vi "HaloDrive.vi"(0 "RobotDriveDevRef 2":T1={"DevStatus"={"status"=FALSE, "code"=0, "source"=""}, "Motors[]"=[], "Square Inputs"=FALSE, "Max Output"=1.0}, 1 "QwikTurnButton":bool, 5 "Left axis value":dbl, 9 "Right axis value":dbl, 11 "error in (no error)":errorcluster, 12 "Sensitivity":dbl) -> (4 "RobotDriveDevRef":T1={"DevStatus"={"status"=FALSE, "code"=0, "source"=""}, "Motors[]"=[], "Square Inputs"=FALSE, "Max Output"=1.0}, 6 "Motor Values":dbl[](array[numeric]), 8 "Left Output":dbl, 10 "Right Output":dbl, 15 "error out":errorcluster)   [LabVIEW 2015]
uses:
  <vilib>/Rock Robotics/WPI/RobotDrive/WPI_RobotDriveDevRef.ctl
  <vilib>/Rock Robotics/WPI/MotorControl/WPI_MotorControlDeviceRef.ctl
  <vilib>/Rock Robotics/WPI/MotorControl/WPI_MotorControlType.ctl
  <vilib>/Rock Robotics/SystemInterfaces/DIO/FPGA_DIOPWMChannel.ctl
  <vilib>/Rock Robotics/WPI/PWM/WPI_PWMDeadband.ctl
  <vilib>/Rock Robotics/WPI/CAN/Jaguar/SubVIs/WPI_CANJaguar_ControlMode.ctl
  <vilib>/Rock Robotics/WPI/CAN/TalonSRX/WPI_CANTalonSRX_APIControlMode.ctl
  <vilib>/Rock Robotics/SystemInterfaces/NetworkCommunication/NetComm_UsageReport_ResourceType.ctl
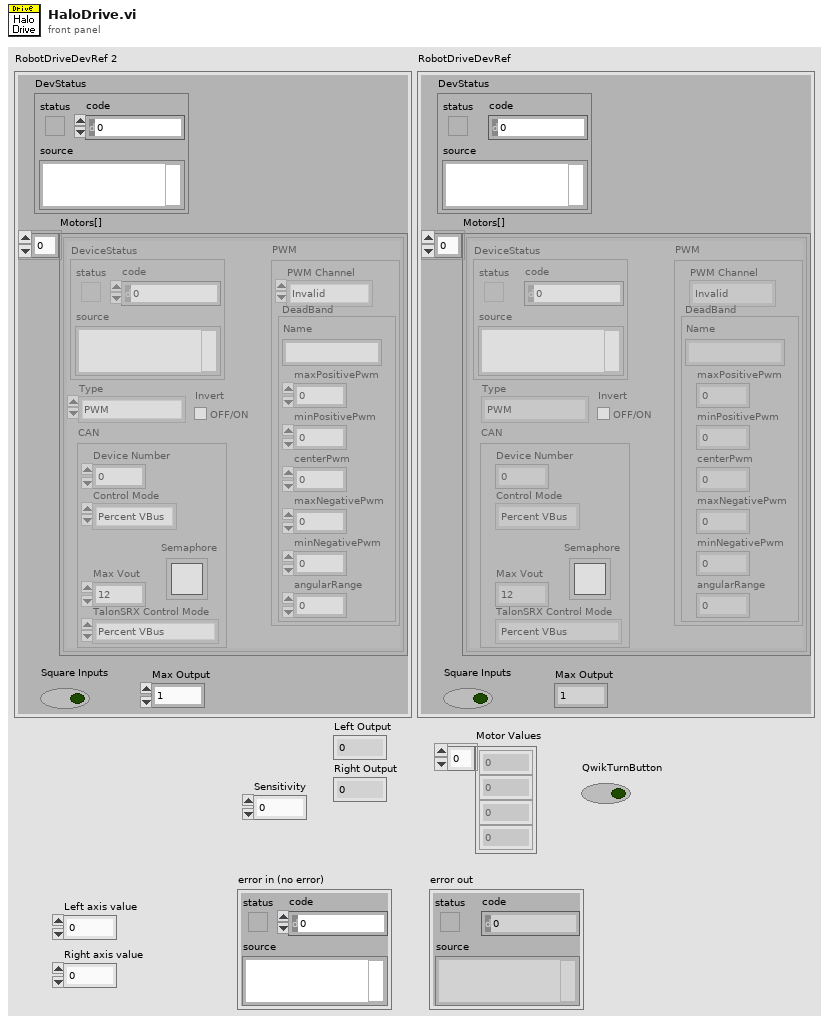
[diagram p1: front panel]
types:
  T1 = typedef "WPI_RobotDriveDevRef.ctl" = cluster{"DevStatus":errorcluster, "Motors[]":T2[], "Square Inputs":bool, "Max Output":dbl}
  T2 = typedef "WPI_MotorControlDeviceRef.ctl" = cluster{"DeviceStatus":errorcluster, "Type":T3, "PWM":cluster{"PWM Channel":T4, "DeadBand":T5}, "CAN":cluster{"Device Number":u8, "Control Mode":T6, "Semaphore":T7, "Max Vout":dbl, "TalonSRX Control Mode":T8}, "Invert":bool}
  T3 = typedef "WPI_MotorControlType.ctl" = enum16{"PWM", "CAN", "CANTalonSRX"}
  T4 = typedef "FPGA_DIOPWMChannel.ctl" = enum8{"PWM 0", "PWM 1", "PWM 2", "PWM 3", "PWM 4", "PWM 5", "PWM 6", "PWM 7", "PWM 8", "PWM 9", "PWM MXP 0", "PWM MXP 1", "PWM MXP 2", "PWM MXP 3", "PWM MXP 4", "PWM MXP 5", "PWM MXP 6", "PWM MXP 7", "PWM MXP 8", "PWM MXP 9", "Invalid"}
  T5 = typedef "WPI_PWMDeadband.ctl" = cluster{"Name":string, "maxPositivePwm":i32, "minPositivePwm":i32, "centerPwm":i32, "maxNegativePwm":i32, "minNegativePwm":i32, "angularRange":u16}
  T6 = typedef "WPI_CANJaguar_ControlMode.ctl" = enum8{"Percent VBus", "Current", "Speed", "Position", "Voltage"}
  T7 = typedef "Semaphore RefNum" = refnum<k1>
  T8 = typedef "WPI_CANTalonSRX_APIControlMode.ctl" = enum8{"Percent VBus", "Speed", "Position", "Slave", "Unchanged / Invalid", "Voltage Compensation", "Current", "Motion Profile"}
  T9 = typedef "NetComm_UsageReport_ResourceType.ctl" = enum8{"Controller", "Module", "Language", "CANPlugin", "Accelerometer", "ADXL345", "AnalogChannel", "AnalogTrigger", "AnalogTriggerOutput", "CANJaguar", "Compressor", "Counter", "Dashboard", "DigitalInput", "DigitalOutput", "DriverStationCIO", "DriverStationEIO", "DriverStationLCD", "Encoder", "GearTooth", "Gyro", "I2C", "Framework", "Jaguar", "Joystick", "Kinect", "KinectStick", "PIDController", "Preferences", "PWM", "Relay", "RobotDrive", "SerialPort", "Servo", "Solenoid", "SPI", "Task", "Ultrasonic", "Victor", "Button", "Command", "AxisCamera", "PCVideoServer", "SmartDashboard", "Talon", "HiTechnicColorSensor", "HiTechnicAccel", "HiTechnicCompass", "SRF08", "AnalogOutput", "Victor SP", "Talon SRX", "CAN Talon SRX", "ADXL362 Accel", "ADXRS450 Gyro", "Rev SPARK", "Mindsensors SD540", "Digital Filter"}
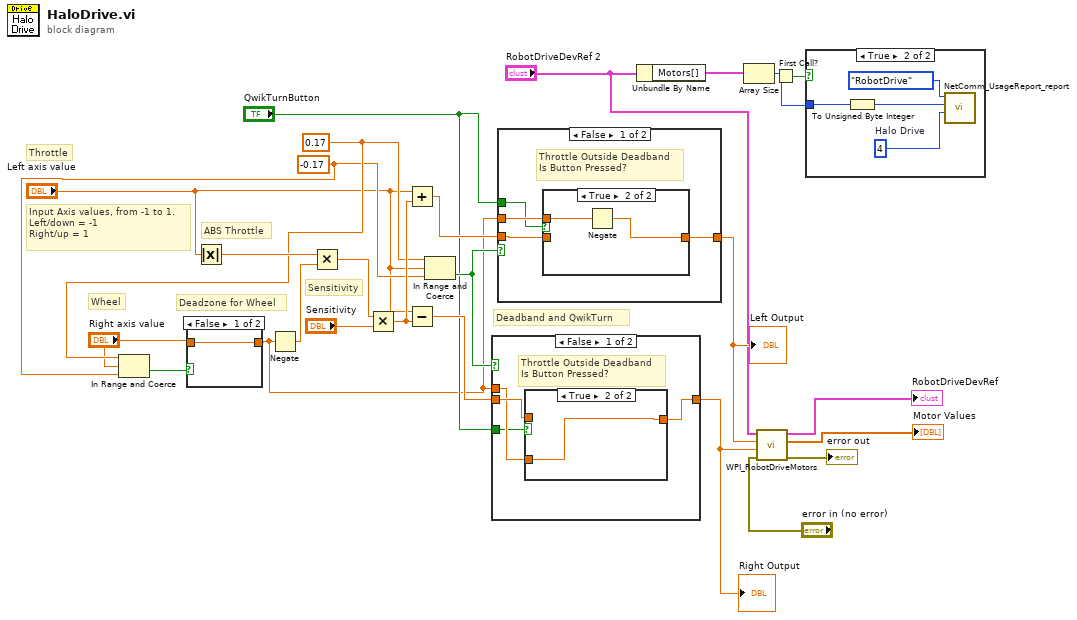
[diagram p0: block diagram]
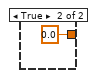
[diagram p2: hidden frame]
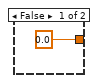
[diagram p5: hidden frame]
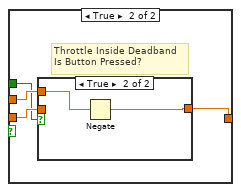
[diagram p7: hidden frame]
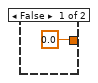
[diagram p8: hidden frame]
diagram:
  w6 = -0.17 ("lower limit")
  w7 = 0.17 ("upper limit")
  # "Deadzone for Wheel"
  # "Deadband and QwikTurn"
  # "Sensitivity"
  # "Wheel"
  # "Throttle"
  # "ABS Throttle"
  # "Input Axis values, from -1 to 1.\nLeft/down = -1\nRight/up = 1"
  n1 = In Range and Coerce(upper limit=w7, x="Right axis value", lower limit=w6) -> (In Range?=w9:bool)  [unwired: 1 out]
  n2 = case shown="False" w9 {
    tunnel: "Right axis value" -> [w26 _]
    tunnel: [w26 0.0 ("Right axis value")] -> w1
    frame False {
    }
    frame True {
    }
  }
  n3 = Absolute Value(x="Left axis value") -> (abs(x)=w18:dbl)
  n4 = Negate(x=w1) -> (-x=w15:dbl)
  n5 = Multiply(x=w18, y=w15) -> (x*y=w17:dbl)
  n6 = Multiply(x=w17, y="Sensitivity") -> (x*y=w16:dbl)
  n7 = Add(x="Left axis value", y=w16) -> (x+y=w10:dbl)
  n8 = Subtract(x="Left axis value", y=w16) -> (x-y=w11:dbl)
  n9 = In Range and Coerce(upper limit=w7, x="Left axis value", lower limit=w6) -> (In Range?=w4:bool)  [unwired: 1 out]
  n10 = case shown="False" w4 {
    tunnel: [w31 w36] -> w13
    tunnel: w11 -> [w30 _]
    tunnel: w1 -> [w29 w35]
    tunnel: "QwikTurnButton" -> [w28 w34]
    frame False {
      # "Throttle Outside Deadband\nIs Button Pressed?"
      n11 = case shown="True" w28 {
        tunnel: w30 -> [w32 _]
        tunnel: [w32 w33] -> w31
        tunnel: w29 -> [_ w33]
        frame False {
        }
        frame True {
        }
      }
    }
    frame True {
      # "Throttle Inside Deadband\nIs Button Pressed?"
      n12 = case shown="True" w34 {
        tunnel: [0.0 w38] -> w36
        tunnel: w35 -> [_ w38]
        frame False {
        }
        frame True {
        }
      }
    }
  }
  "Right Output" <- w13
  n13 = case shown="False" w4 {
    tunnel: w10 -> [w41 w47]
    tunnel: [w42 w48] -> w14
    tunnel: w1 -> [w40 w49]
    tunnel: "QwikTurnButton" -> [w39 w46]
    frame False {
      # "Throttle Outside Deadband\nIs Button Pressed?"
      n14 = case shown="True" w39 {
        tunnel: w41 -> [w43 _]
        tunnel: [w43 w44] -> w42
        tunnel: w40 -> [_ w45]
        frame False {
        }
        frame True {
          n15 = Negate(x=w45) -> (-x=w44:dbl)
        }
      }
    }
    frame True {
      # "Throttle Inside Deadband\nIs Button Pressed?"
      n16 = case shown="True" w46 {
        tunnel: w49 -> [_ w52]
        tunnel: [0.0 w51] -> w48
        tunnel: w47 -> [_ _]
        frame False {
        }
        frame True {
          n17 = Negate(x=w52) -> (-x=w51:dbl)
        }
      }
    }
  }
  "Left Output" <- w14
  n18 = Unbundle By Name("RobotDriveDevRef 2") -> ("Motors[]"=w21:T2[])
  n19 = Array Size(array=w21) -> (size(s)=w20:i32)
  n20 = call <vilib>:"WPI_RobotDriveMotors.vi"("error in (no error)"="error in (no error)", "RightSpeed"=w13, "LeftSpeed"=w14, "RobotDriveDevRef"="RobotDriveDevRef 2") -> ("error out"=→"error out":errorcluster, "Motor Values"=→"Motor Values":dbl[], "RobotDriveDevRef"=→"RobotDriveDevRef":T1)  [unwired: 5 out]
  n21 = First Call?() -> (First Call?: T/F=w22:bool)
  n22 = case shown="True" w22 {
    tunnel: w20 -> [_ w55]
    frame False {
    }
    frame True {
      w53 = u8 4  # Halo Drive
      n23 = To Unsigned Byte Integer(number=w55) -> (unsigned 8bit integer=w54:u8)
      n24 = call <vilib>:"NetComm_UsageReport_report.vi"("Context"=w53, "Instance Number"=w54, "Resource Type"=NetComm_UsageReport_ResourceType."RobotDrive") -> ()  [unwired: 9 in]
    }
  }
